vi "Thread.vi"(8 "error in (no error)":errorcluster, 11 "This":refnum<class "WebSocket.lvclass">) -> (0 "error out":errorcluster, 3 "WebSocket out":refnum<class "WebSocket.lvclass">)   [LabVIEW 2023, in "WebSocket.lvclass"]
uses:
  WebSocket.lvclass
  protected/WebSocket Packet.ctl
  private/Fixed Header.ctl
  private/OpCode.ctl
  Log/Log_Facilities.ctl
  Log/Log.lvclass
panel:
  out "Packet In Process":T1
  out "Last Rx Packet":string
  out "Data":T1
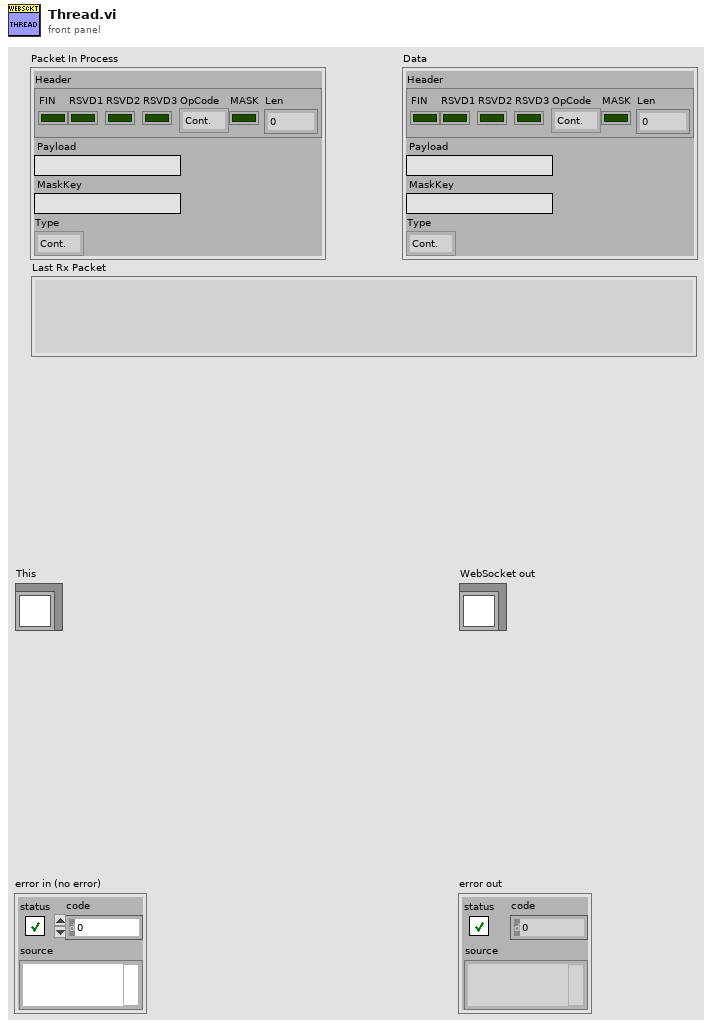
[diagram p1: front panel]
types:
  T1 = typedef "WebSocket.lvclass/WebSocket Packet.ctl" = cluster{"Header":T2, "Payload":string, "MaskKey":string, "Type":T3}
  T2 = typedef "WebSocket.lvclass/Fixed Header.ctl" = cluster{"FIN":bool, "RSVD1":bool, "RSVD2":bool, "RSVD3":bool, "OpCode":T3, "MASK":bool, "Len":u8}
  T3 = typedef "WebSocket.lvclass/OpCode.ctl" = enum16{"Cont.", "Text", "Binary", "NonCtl3", "NonCtl4", "NonCtl5", "NonCtl6", "NonCtl7", "Close", "Ping", "Pong", "Rsvd11", "Rsvd12", "Rsvd13", "Rsvd14", "Rsvd15"}
  T4 = typedef "Log.lvclass/Log_Facilities.ctl" = string
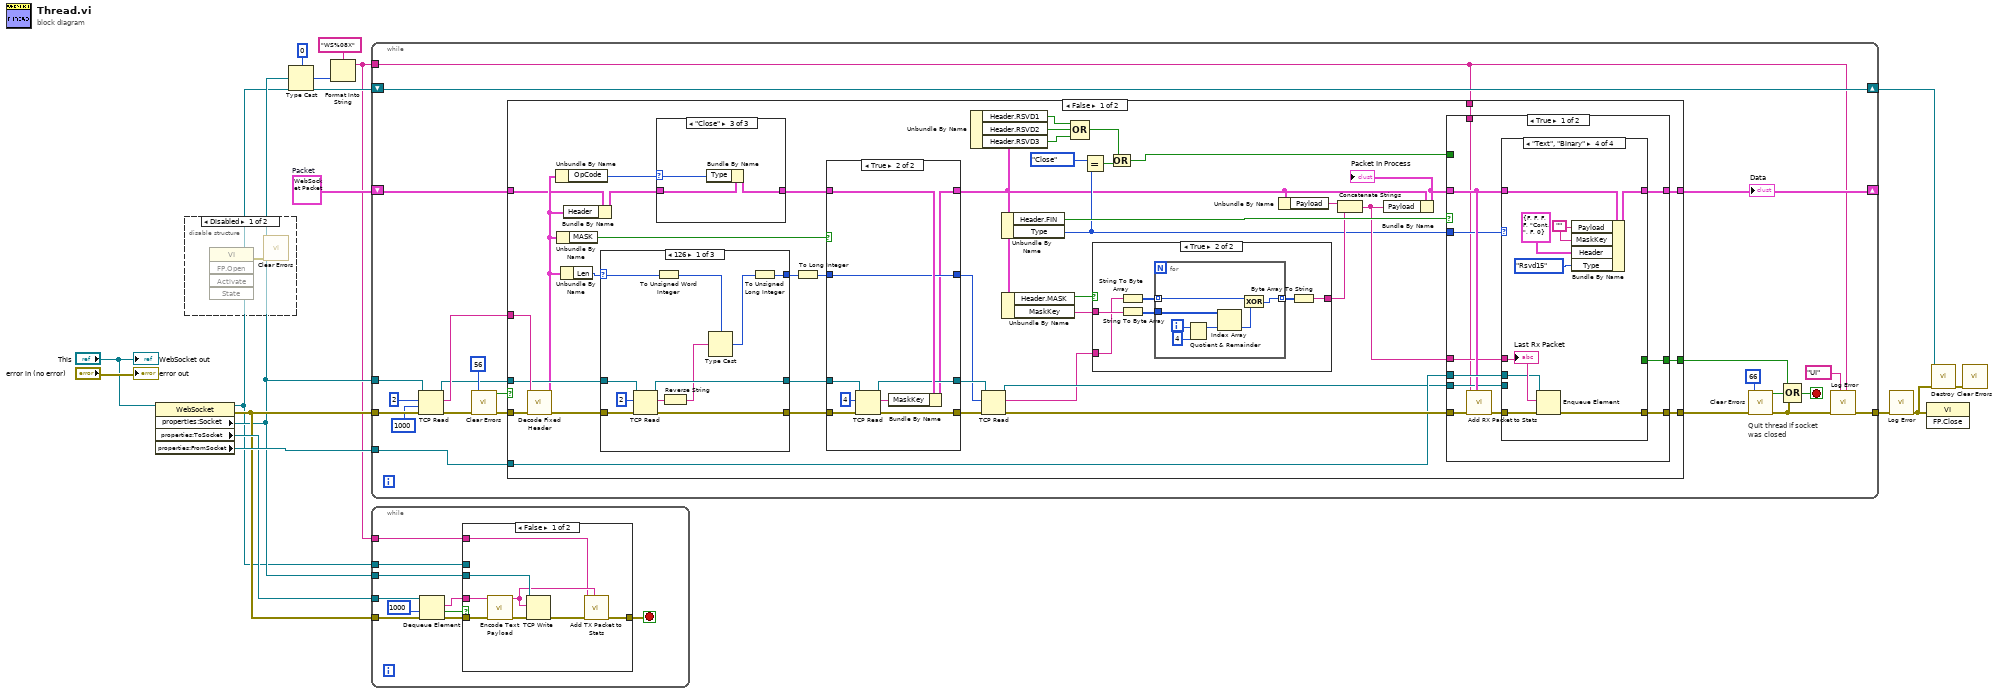
[diagram p0: block diagram]
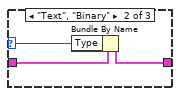
[diagram p5: hidden frame]
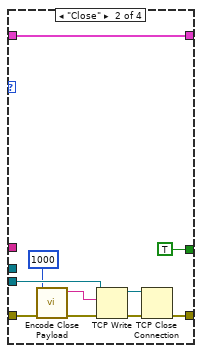
[diagram p8: hidden frame]
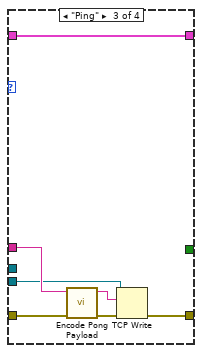
[diagram p9: hidden frame]
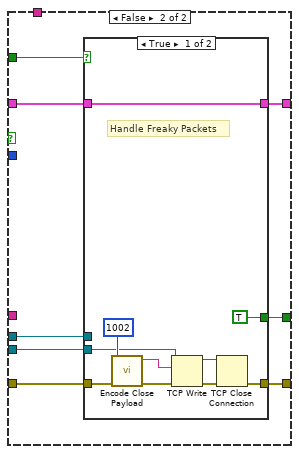
[diagram p10: hidden frame]
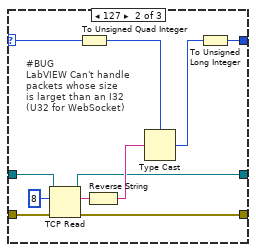
[diagram p13: hidden frame]
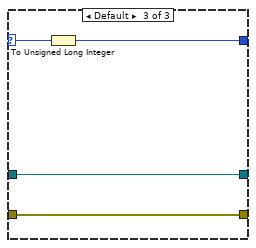
[diagram p14: hidden frame]
diagram:
  w14 = T1 {"Header"={"FIN"=FALSE, "RSVD1"=FALSE, "RSVD2"=FALSE, "RSVD3"=FALSE, "OpCode"=enum."Cont.", "MASK"=FALSE, "Len"=0}, "Payload"="", "MaskKey"="", "Type"=enum."Cont."}  # Packet
  n1 = property class="WebSocket"(reference="This") -> (reference out=w2:refnum<class "WebSocket.lvclass">, error out=w10:errorcluster, "properties:Socket"=w5:refnum<k5>, "properties:ToSocket"=w11:refnum<queue>, "properties:FromSocket"=w13:refnum<queue>)  [unwired: 1 in]
  n2 = disable-structure shown="Disabled" {
    frame Disabled {
      n3 = invoke class="VI" method="FP.Open"() -> (error out=w17:errorcluster)  [unwired: 5 in, 4 out]
      n4 = call <vilib>:"Clear Errors.vi"("error in (no error)"=w17) -> ()  [unwired: 5 in, 2 out]
    }
    frame Enabled {
    }
  }
  n5 = Type Cast(type=u32 0 ("input 1"), x=w5) -> (*(type *) &x=w3:u32)
  n6 = Format Into String(format string="WS%08X", w3) -> (resulting string=w1:string)  [unwired: 2 in, 1 out]
  n7 = while {
    tunnel: w10 -> [w40]
    shift-right: [w19] -> w8
    shift-left: w2 -> [w19]
    tunnel: [w22] -> w12
    tunnel: w5 -> [w39]
    shift-right: [w24] -> _
    shift-left: w14 -> [w38]
    tunnel: w13 -> [w37]
    tunnel: w1 -> [w18]
    stop <- w36 stop-if-true
    # "Quit thread if socket\nwas closed"
    n8 = TCP Read(connection ID=w39, bytes to read=2, error in (no error)=w40, 9:1000 ("timeout ms (25000)")) -> (connection ID out=w26:refnum<k5>, data out=w28:string, error out=w32:errorcluster)  [unwired: 1 in]
    n9 = call <vilib>:"Clear Errors.vi"("error in (no error)"=w32, "specific error code to clear (0: all)"=56) -> ("error out"=w30:errorcluster, "specific error cleared?"=w29:bool)  [unwired: 4 in]
    n10 = case shown="False" w29 {
      tunnel: w28 -> [w81 _]
      tunnel: w30 -> [w82 w203]
      tunnel: [w64 w203] -> w20
      tunnel: w26 -> [w78 _]
      tunnel: w38 -> [w58 w202]
      tunnel: [w69 w202] -> w24
      tunnel: w37 -> [w65 _]
      tunnel: [w53 _] -> w35
      tunnel: w18 -> [w41 _]
      frame False {
        n11 = call "Decode Fixed Header.vi"("error in (no error)"=w82, "String"=w81) -> ("error out"=w80:errorcluster, "Fixed Header"=w59:T2)  [unwired: 8 in]
        n12 = Unbundle By Name(w59) -> ("OpCode"=w57:T3)
        n13 = Unbundle By Name(w59) -> ("MASK"=w76:bool)
        n14 = Unbundle By Name(w59) -> ("Len"=w79:u8)
        n15 = Bundle By Name(cluster=w58, "Header"=w59) -> (w56:T1)
        n16 = case shown="126" w79 {
          selector: w79 -> [w179 w192 w201]
          tunnel: [w176 w189 w198] -> w74
          tunnel: w78 -> [w185 w188 w199]
          tunnel: w80 -> [w184 w196 w200]
          tunnel: [w186 w197 w200] -> w77
          tunnel: [w183 w187 w199] -> w75
          frame 126 {
            n17 = TCP Read(connection ID=w185, bytes to read=2, error in (no error)=w184) -> (connection ID out=w183:refnum<k5>, data out=w182:string, error out=w186:errorcluster)  [unwired: 2 in]
            n18 = To Unsigned Word Integer(number=w179) -> (unsigned 16bit integer=w177:u16)
            n19 = Reverse String(1:w182) -> (0:w180:string)
            n20 = Type Cast(type=w177, x=w180) -> (*(type *) &x=w178:u16)
            n21 = To Unsigned Long Integer(number=w178) -> (unsigned 32bit integer=w176:u32)
          }
          frame 127 {
            # "#BUG\nLabVIEW Can't handle\npackets whose size\nis larget than an I32\n(U32 for WebSocket)"
            n22 = TCP Read(connection ID=w188, bytes to read=8, error in (no error)=w196) -> (connection ID out=w187:refnum<k5>, data out=w195:string, error out=w197:errorcluster)  [unwired: 2 in]
            n23 = To Unsigned Quad Integer(1:w192) -> (0:w190:u64)
            n24 = Reverse String(1:w195) -> (0:w193:string)
            n25 = Type Cast(type=w190, x=w193) -> (*(type *) &x=w191:u64)
            n26 = To Unsigned Long Integer(number=w191) -> (unsigned 32bit integer=w189:u32)
          }
          frame Default {
            n27 = To Unsigned Long Integer(number=w201) -> (unsigned 32bit integer=w198:u32)
          }
        }
        n28 = case shown="\"Close\"" w57 {
          selector: w57 -> [_ w84 w87]
          tunnel: w56 -> [w83 w85 w88]
          tunnel: [w83 w86 w89] -> w55
          frame Default {
          }
          frame "Text", "Binary" {
            n29 = Bundle By Name(cluster=w85, "Type"=w84) -> (w86:T1)
          }
          frame "Close" {
            n30 = Bundle By Name(cluster=w88, "Type"=w87) -> (w89:T1)
          }
        }
        n31 = To Long Integer(number=w74) -> (32bit integer=w43:i32)
        n32 = case shown="True" w76 {
          tunnel: w55 -> [w166 w172]
          tunnel: [w166 w167] -> w49
          tunnel: w77 -> [w164 w175]
          tunnel: w75 -> [w165 w174]
          tunnel: [w165 w171] -> w72
          tunnel: [w164 w170] -> w73
          tunnel: [w163 w168] -> w71
          tunnel: w43 -> [w163 w168]
          frame False {
          }
          frame True {
            n33 = TCP Read(connection ID=w174, bytes to read=4, error in (no error)=w175) -> (connection ID out=w171:refnum<k5>, data out=w169:string, error out=w170:errorcluster)  [unwired: 2 in]
            n34 = Bundle By Name(cluster=w172, "MaskKey"=w169) -> (w167:T1)
          }
        }
        n35 = Unbundle By Name(w49) -> ("Header.RSVD1"=w47:bool, "Header.RSVD2"=w48:bool, "Header.RSVD3"=w46:bool)
        n36 = TCP Read(connection ID=w72, bytes to read=w71, error in (no error)=w73) -> (connection ID out=w54:refnum<k5>, data out=w42:string, error out=w66:errorcluster)  [unwired: 2 in]
        n37 = Unbundle By Name(w49) -> ("Header.FIN"=w70:bool, "Type"=w52:T3)
        n38 = Unbundle By Name(w49) -> ("Header.MASK"=w68:bool, "MaskKey"=w67:string)
        n39 = Compound Arithmetic op=OR(w47, w48, w46) -> (w45:bool)
        n40 = Equal?(x=OpCode."Close", y=w52) -> (x = y?=w50:bool)
        n41 = case shown="True" w68 {
          tunnel: w67 -> [_ w93]
          tunnel: [w90 w92] -> w62
          tunnel: w42 -> [w90 w91]
          frame False {
          }
          frame True {
            n42 = String To Byte Array(string=w91) -> (unsigned byte array=w96:u8[])
            n43 = String To Byte Array(string=w93) -> (unsigned byte array=w95:u8[])
            n44 = for {
              tunnel: w96 -> [w98] mode=indexing
              tunnel: w95 -> [w100]
              tunnel: [w97] -> w94 mode=indexing
              i -> [w103]
              n45 = Quotient & Remainder(x=w103, y=4) -> (x-y*floor(x/y)=w101:i32)  [unwired: 1 out]
              n46 = Index Array(array=w100, index=w101) -> (element=w99:u8)
              n47 = Exclusive Or(1:w99, 2:w98) -> (0:w97:u8)
            }
            n48 = Byte Array To String(unsigned byte array=w94) -> (string=w92:string)
          }
        }
        n49 = Or(x=w45, y=w50) -> (x .or. y?=w44:bool)
        n50 = Unbundle By Name(w49) -> ("Payload"=w63:string)
        n51 = Concatenate Strings(w63, w62) -> (w61:string)
        n52 = Bundle By Name(cluster=w49, "Payload"=w61) -> (w60:T1)
        "Packet In Process" <- w60
        n53 = case shown="True" w70 {
          tunnel: [w114 w143] -> w69
          tunnel: w60 -> [w111 w148]
          tunnel: w66 -> [w105 w147]
          tunnel: w65 -> [w112 w146]
          tunnel: [w113 w144] -> w64
          tunnel: w61 -> [w110 _]
          tunnel: w52 -> [w109 _]
          tunnel: w54 -> [w108 w145]
          tunnel: [w107 w149] -> w53
          tunnel: w44 -> [_ w150]
          tunnel: w41 -> [w104 _]
          frame True {
            n54 = call "Add RX Packet to Stats.vi"("Packet"=w111, "error in (no error)"=w105, "Name"=w104) -> ("error out"=w106:errorcluster)  [unwired: 8 in]
            n55 = case shown="\"Text\", \"Binary\"" w109 {
              tunnel: [w116 w126 w133 w142] -> w114
              tunnel: w106 -> [w115 w125 w131 w141]
              tunnel: [w115 w123 w129 w140] -> w113
              tunnel: w112 -> [_ _ _ w134]
              tunnel: w111 -> [w116 w126 w133 w135]
              tunnel: w110 -> [_ _ w128 w139]
              tunnel: w108 -> [_ w120 w127 _]
              tunnel: [_ TRUE _ _] -> w107
              frame Default {
              }
              frame "Close" {
                n56 = call "Encode Close Payload.vi"("error in (no error)"=w125, "Code"=u32 1000) -> ("error out"=w121:errorcluster, "Packet"=w118:string)  [unwired: 8 in]
                n57 = TCP Write(connection ID=w120, data in=w118, error in (no error)=w121) -> (connection ID out=w119:refnum<k5>, error out=w122:errorcluster)  [unwired: 1 in, 1 out]
                n58 = TCP Close Connection(connection ID=w119, error in (no error)=w122) -> (error out=w123:errorcluster)  [unwired: 1 in, 1 out]
              }
              frame "Ping" {
                n59 = call "Encode Pong Payload.vi"("error in (no error)"=w131, "Payload"=w128) -> ("error out"=w130:errorcluster, "Packet"=w132:string)  [unwired: 8 in]
                n60 = TCP Write(connection ID=w127, data in=w132, error in (no error)=w130) -> (error out=w129:errorcluster)  [unwired: 1 in, 2 out]
              }
              frame "Text", "Binary" {
                w138 = ""
                n61 = Enqueue Element(queue=w134, element=w139, error in (no error)=w141) -> (error out=w140:errorcluster)  [unwired: 1 in, 2 out]
                n62 = Bundle By Name(cluster=w135, "Payload"=w138, "MaskKey"=w138, "Header"=T2 {"FIN"=FALSE, "RSVD1"=FALSE, "RSVD2"=FALSE, "RSVD3"=FALSE, "OpCode"=enum."Cont.", "MASK"=FALSE, "Len"=0}, "Type"=OpCode."Rsvd15") -> (w142:T1)
                "Last Rx Packet" <- w139
              }
            }
          }
          frame False {
            n63 = case shown="True" w150 {
              tunnel: [w160 w162] -> w143
              tunnel: w147 -> [w153 w161]
              tunnel: [w151 w161] -> w144
              tunnel: w146 -> [_ _]
              tunnel: w148 -> [w160 w162]
              tunnel: w145 -> [w152 _]
              tunnel: [TRUE _] -> w149
              frame True {
                # "Handle Freaky Packets"
                n64 = call "Encode Close Payload.vi"("error in (no error)"=w153, "Code"=u32 1002) -> ("error out"=w157:errorcluster, "Packet"=w155:string)  [unwired: 8 in]
                n65 = TCP Write(connection ID=w152, data in=w155, error in (no error)=w157) -> (connection ID out=w156:refnum<k5>, error out=w158:errorcluster)  [unwired: 1 in, 1 out]
                n66 = TCP Close Connection(connection ID=w156, error in (no error)=w158) -> (error out=w151:errorcluster)  [unwired: 1 in, 1 out]
              }
              frame False {
              }
            }
          }
        }
      }
      frame True {
      }
    }
    "Data" <- w24
    n67 = call <vilib>:"Clear Errors.vi"("error in (no error)"=w20, "specific error code to clear (0: all)"=66) -> ("error out"=w23:errorcluster, "specific error cleared?"=w25:bool)  [unwired: 4 in]
    n68 = Compound Arithmetic op=OR(w35, w25, w23) -> (w36:bool)
    n69 = call "Log Error.vi"("Context"=w18, "Facility (default)"=T4 "UI", "error in (no error)"=w23) -> ("error out"=w22:errorcluster)  [unwired: 8 in]
  }
  n70 = while {
    tunnel: w11 -> [w210]
    tunnel: w5 -> [w209]
    tunnel: w10 -> [w208]
    tunnel: w2 -> [w205]
    tunnel: w1 -> [w204]
    stop <- w207 stop-if-true
    n71 = Dequeue Element(queue=w210, timeout in ms (-1)=1000, error in (no error)=w208) -> (element=w211:string, timed out?=w213:bool, error out=w212:errorcluster)  [unwired: 1 out]
    n72 = case shown="False" w213 {
      tunnel: w212 -> [w220 w222]
      tunnel: [w216 w222] -> w207
      tunnel: w211 -> [w219 _]
      tunnel: w209 -> [w221 _]
      tunnel: w205 -> [_ _]
      tunnel: w204 -> [w214 _]
      frame False {
        n73 = call "Encode Text Payload.vi"("error in (no error)"=w220, "Text"=w219) -> ("error out"=w218:errorcluster, "Packet"=w215:string)  [unwired: 8 in]
        n74 = TCP Write(connection ID=w221, data in=w215, error in (no error)=w218) -> (error out=w217:errorcluster)  [unwired: 1 in, 2 out]
        n75 = call "Add TX Packet to Stats.vi"("Packet"=w215, "error in (no error)"=w217, "Name"=w214) -> ("error out"=w216:errorcluster)  [unwired: 8 in]
      }
      frame True {
      }
    }
  }
  n76 = call "Log Error.vi"("error in (no error)"=w12) -> ("error out"=w9:errorcluster)  [unwired: 10 in]
  n77 = invoke class="VI" method="FP.Close"(error in=w9) -> ()  [unwired: 2 in, 3 out]
  n78 = call-dynamic "Destroy.vi"("error in (no error)"=w9, "reference in"=w8) -> ("error out"=w7:errorcluster)  [unwired: 8 in, 1 out]
  n79 = call <vilib>:"Clear Errors.vi"("error in (no error)"=w7) -> ()  [unwired: 5 in, 2 out]
  "error out" <- "error in (no error)"
  "WebSocket out" <- "This"
